vi "PH_Cont-601k_PSU.PC Write PSDB.vi"(0 "i ref in":refnum<vi>, 5 "error IO":errorcluster) -> (14 "i ref out":refnum<vi>, 19 "error out":errorcluster)   [LabVIEW 2014]
doc: "This is the proc case which sets the data to be written to the to the PHELIX shot data base."
uses:
  PH_PSDBWriter/PH_PSDBWriter.2D dataset.ctl
  User/Eisenbarth/PSDB/PSDB_AxisDescription.ctl
  <vilib>/vision/Image Controls.llb/IMAQ Image.ctl
  PH_Cont-601k_PSU.lvlib
  PH_PSDBWriter/PH_PSDBWriter.lvlib
panel:
  in  "axis description":T1
  in  "2D data":T2
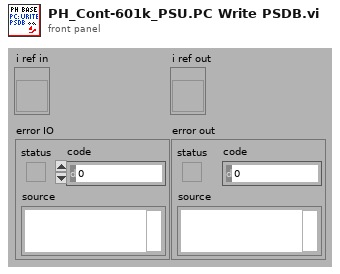
[diagram p1: front panel]
types:
  T1 = typedef "PSDB_AxisDescription.ctl" = cluster{"x axis label":string, "y axis label":string, "x axis unit":string, "y axis unit":string}
  T2 = typedef "PH_PSDBWriter.lvlib/PH_PSDBWriter.2D dataset.ctl" = cluster{"name":string, "data":dbl[][], "axis description":T1}
  T3 = typedef "IMAQ Image.ctl" = refnum<image>
  T4 = typedef "PH_Cont-601k_PSU.lvlib/PH_Cont-601k_PSU.i attribute.ctl" = cluster{"GUI Refs":cluster{"Dummy":refnum<vi>, "Delete":refnum<vi>, "Status":refnum<vi>}, "Status":cluster{"Service ID":i32, "Device Status":T5}, "Related Device 1":cluster{"Instancename":string, "Device Status":T5, "linked?":bool}, "Related Device 2":cluster{"Instancename":string, "linked?":bool}, "GUI Manager Path":string}
  T5 = typedef "Status.ctl" = i16
  T6 = typedef "PH_PSDBWriter.lvlib/PH_PSDBWriter.Boolean dataset.ctl" = cluster{"name":string, "data":bool, "unit":string}
  T7 = typedef "PH_PSDBWriter.lvlib/PH_PSDBWriter.Image dataset.ctl" = cluster{"name":string, "data":T3, "unit":string}
  T8 = typedef "PH_PSDBWriter.lvlib/PH_PSDBWriter.Numeric dataset.ctl" = cluster{"name":string, "data":dbl, "unit":string}
  T9 = typedef "PH_PSDBWriter.lvlib/PH_PSDBWriter.String dataset.ctl" = cluster{"name":string, "data":string, "unit":string}
  T10 = typedef "PH_PSDBWriter.lvlib/PH_PSDBWriter.PSDB Dataset.ctl" = cluster{"Version":i32, "2D data Input":T2[], "Boolean Input":T6[], "Image Input":T7[], "Numeric Input":T8[], "String Input":T9[]}
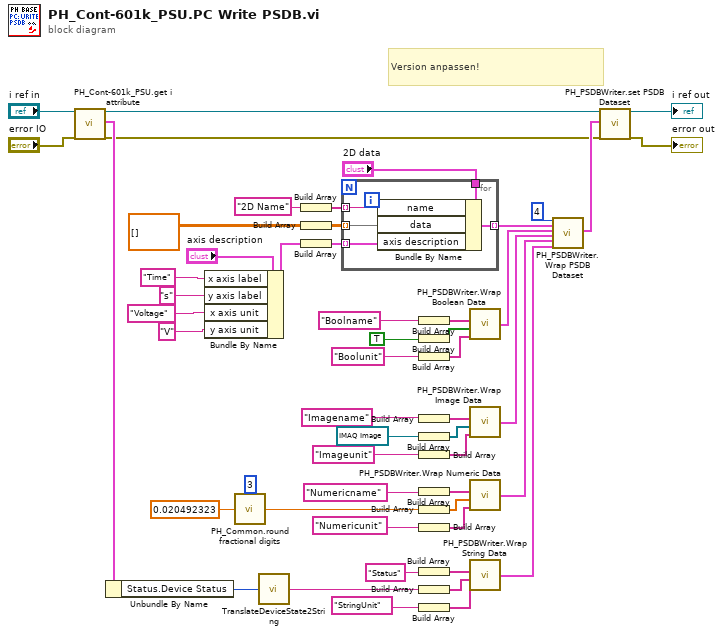
[diagram p0: block diagram]
diagram:
  # "Version anpassen!"
  n1 = call "PH_Cont-601k_PSU.get i attribute.vi"("i ref in"="i ref in", "error in (no error)"="error IO") -> ("i ref out"=w17:refnum<vi>, "i attribute"=w51:T4, "error out"=w14:errorcluster)  [unwired: 15 in]
  n2 = Unbundle By Name(w51) -> ("Status.Device Status"=w50:T5)
  n3 = Bundle By Name(cluster="axis description", "x axis label"="Time", "y axis label"="s", "x axis unit"="Voltage", "y axis unit"="V") -> (w28:T1)
  n4 = call "PH_Common.round fractional digits.vi"("Input"=0.020492323, "Position (1)"=i16 3) -> ("round Output"=w42:dbl)
  n5 = call "TranslateDeviceState2String.vi"("Device Status"=w50) -> ("Device Status as string"=w49:string)
  n6 = Build Array("2D Name") -> (w34:string[])
  n7 = Build Array(dbl[][] [] ("data")) -> (w35:dbl[][][])
  n8 = Build Array(w28) -> (w33:T1[])
  n9 = for {
    tunnel: "2D data" -> [w58]
    tunnel: [w57] -> w1 mode=indexing
    tunnel: w35 -> [w55] mode=indexing
    tunnel: w34 -> [w56] mode=indexing
    tunnel: w33 -> [w54] mode=indexing
    n10 = Bundle By Name(cluster=w58, "name"=w56, "data"=w55, "axis description"=w54) -> (w57:T2)
  }
  n11 = Build Array("Boolname") -> (w13:string[])
  n12 = Build Array(TRUE) -> (w12:bool[])
  n13 = Build Array("Boolunit") -> (w11:string[])
  n14 = Build Array("Imagename") -> (w10:string[])
  n15 = Build Array(T3 refnum ("data")) -> (w9:T3[])
  n16 = Build Array("Imageunit") -> (w8:string[])
  n17 = Build Array("Numericname" ("name")) -> (w7:string[])
  n18 = Build Array(w42) -> (w6:dbl[])
  n19 = Build Array("Numericunit" ("unit")) -> (w5:string[])
  n20 = Build Array("Status" ("name")) -> (w4:string[])
  n21 = Build Array(w49) -> (w3:string[])
  n22 = Build Array("StringUnit" ("unit")) -> (w2:string[])
  n23 = call "PH_PSDBWriter.Wrap Boolean Data.vi"("Unit Array"=w11, "Data Array"=w12, "Name Array"=w13) -> ("PSDB Boolean Data Array"=w19:T6[])  [unwired: 1 in]
  n24 = call "PH_PSDBWriter.Wrap Image Data.vi"("Unit Array"=w8, "Data Arrray"=w9, "Name Array"=w10) -> ("PSDB Image Data Array"=w20:T7[])  [unwired: 1 in]
  n25 = call "PH_PSDBWriter.Wrap Numeric Data.vi"("Unit Array"=w5, "Data Array"=w6, "Name Array"=w7) -> ("PSDB Numeric Data Array"=w21:T8[])  [unwired: 1 in]
  n26 = call "PH_PSDBWriter.Wrap String Data.vi"("Unit Array"=w2, "Data Array"=w3, "Name Array"=w4) -> ("PSDB String Data Array"=w23:T9[])  [unwired: 1 in]
  n27 = call "PH_PSDBWriter.Wrap PSDB Dataset.vi"("Version"=4, "2D data Input"=w1, "Boolean Input"=w19, "Image Input"=w20, "Numeric Input"=w21, "String Input"=w23) -> ("PSDB Dataset"=w22:T10)  [unwired: 13 in]
  n28 = call "PH_PSDBWriter.set PSDB Dataset.vi"("VI in"=w17, "PSDB Dataset"=w22, "error in (no error)"=w14) -> ("VI out"=→"i ref out":refnum<vi>, "error out"=→"error out":errorcluster)  [unwired: 15 in]
